vi "PrintMenu.vi"(8 "Error In":errorcluster, 10 "Iter":refnum<class "IEnumerable.lvclass">, 11 "reference in":refnum<class "Client.lvclass">) -> (0 "Error Out":errorcluster, 3 "reference out":refnum<class "Client.lvclass">)   [LabVIEW 2020, in "Client.lvclass"]
uses:
  Client.lvclass
  IEnumerable_interface/IEnumerable.lvclass
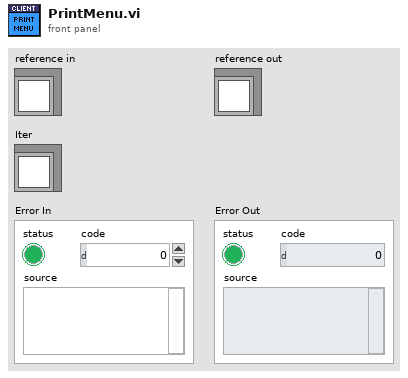
[diagram p1: front panel]
types:
  T1 = typedef "Client.lvclass/ObjectAttributes.ctl" = cluster{"_breakfast":refnum<class "IEnumerable.lvclass">, "_dinner":refnum<class "IEnumerable.lvclass">}
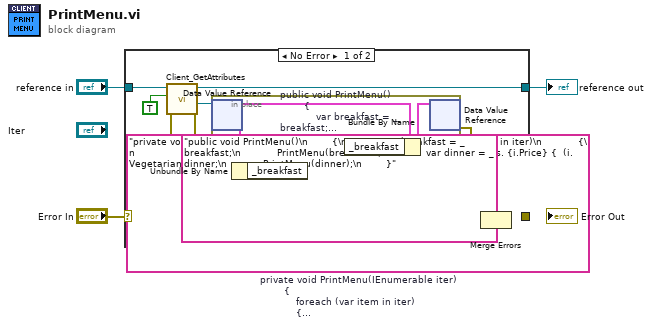
[diagram p0: block diagram]
diagram:
  (unwired) "private void PrintMenu(IEnumerable iter)\n        {\n            foreach (var item in iter)\n            {\n                var i = (Menu)item;\n                Console.WriteLine($\"{i.Name}  Rs. {i.Price} {  (i.Vegetarian ? \"*\" : \"x\") } \\n {i.Description} \");\n\n            }\n        }"  # private void PrintMenu(IEnumerable iter)         {             foreach (var item in iter)             {                 var i = (Menu)item;                 Console.WriteLine($"{i.Name}  Rs. {i.Price} {  (i.Vegetarian ? "*" : "x") } \n {i.Description} ");              }         }
  (unwired) "public void PrintMenu()\n        {\n            var breakfast = _breakfast;\n            PrintMenu(breakfast);\n            var dinner = _dinner;\n            PrintMenu(dinner);\n        }"  # public void PrintMenu()         {             var breakfast = _breakfast;             PrintMenu(breakfast);             var dinner = _dinner;             PrintMenu(dinner);         }
  n1 = case shown="No Error" "Error In" {
    selector: "Error In" -> [w11 w16]
    tunnel: [w8 w16] -> w3
    tunnel: [w9 w15] -> w1
    tunnel: "reference in" -> [w12 w15]
    frame No Error {
      n2 = call "Client_GetAttributes.vi"("error in (no error)"=w11, "OnlyGetDvrReference(False)"=TRUE, "reference in"=w12) -> ("error out"=w6:errorcluster, "DataRef"=w7:refnum<data-value>, "reference out"=w9:refnum<class "Client.lvclass">)  [unwired: 5 in, 1 out]
      n3 = in-place {
        n4 = in-place-dvr #1(w7) -> (w13:T1)  [unwired: 1 out]
        n5 = Unbundle By Name(w13) -> ()  [unwired: 1 out]
        n6 = Bundle By Name(cluster=w13) -> (w14:T1)  [unwired: 1 in]
        n7 = in-place-dvr #1(w14) -> (w10:errorcluster)  [unwired: 1 out]
      }
      n8 = Merge Errors(w6, w10) -> (w8:errorcluster)
    }
    frame Error {
    }
  }
  "Error Out" <- w3
  "reference out" <- w1
